vi "UpdateOutToFileFromFile.vi"(8 "ErrorArray In":errorcluster[](array[cluster]), 10 "TestFileRef In":T1, 11 "Bus In":refnum<class "Bus.lvclass">) -> (0 "ErrorArray Out":errorcluster[](array[cluster]), 2 "refnum out":T1, 3 "Bus Out":refnum<class "Bus.lvclass">)   [LabVIEW 2017, in "Bus_class.lvlib" / "Bus.lvclass"]
uses:
  Bus.lvclass
  <vilib>/Utility/config.llb/Config Data RefNum.ctl
  Modules/OutputToFilePlugins/OutputToFileBasePlugin/Typedefs/PmuCfgOpt.ctl
  TypeDefs/clBusData.ctl
  FrontPanel/TypeDefs/clEventConfig.ctl
  Modules/PmuImpairPlugins/PmuImpairPluginBase_class/TypeDefs/clImpairConfig.ctl
  Modules/EventPlugins/EventPluginBaseClass/TypeDefs/clEvtReportArray.ctl
  Modules/EventPlugins/EventPluginBaseClass/TypeDefs/clEvtReport.ctl
  Modules/EventPlugins/EventPluginBaseClass/TypeDefs/dblEvtSignalArray.ctl
  Modules/NetworkImpairmentModule/PublicAPI/Arguments/Broadcasts/dblNetworkTime.ctl
  Modules/NetworkImpairmentModule/PublicAPI/Arguments/Broadcasts/dblPktLoss.ctl
  Modules/FlagImpairModule/PublicAPI/Arguments/Broadcasts/ui32FlagImpairmentArray.ctl
  Modules/OutputToFilePlugins/OutputToFileBasePlugin/OutputToFileBasePlugin.lvclass
  Modules/FlagImpairModule/FlagImpairModule.lvlib
  Modules/NetworkImpairmentModule/NetworkImpairmentModule.lvlib
  Modules/EventPlugins/EventPluginBaseClass/EventPluginBaseClass.lvclass
  Modules/PmuImpairPlugins/PmuImpairPluginBase_class/PmuImpairPluginBase.lvclass
  Framework.lvlib
  <userlib>/NIST/NISTErrorLib/NISTErrorLib.lvlib
  <vilib>/Utility/config.llb/NI_LVConfig.lvlib
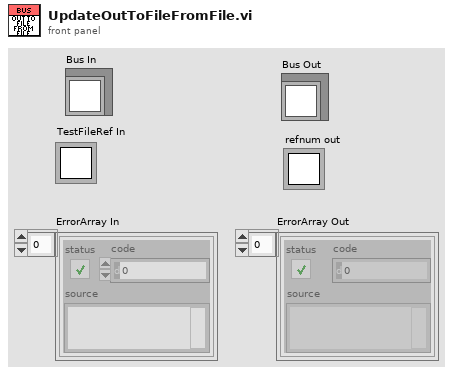
[diagram p1: front panel]
types:
  T1 = typedef "NI_LVConfig.lvlib/Config Data RefNum.ctl" = refnum<k1>
  T2 = typedef "Bus_class.lvlib/Bus.lvclass/clBusData.ctl" = cluster{"BusNumber":u8, "EvtPluginINIFilePath":path, "EvtParams":string[][], "EvtConfig":T3, "Start Time":dbl, "End Time":dbl, "PmuImpairPluginINIFilePath":path, "PmuImpairParams ":string[][], "PmuImpairConfig":T4, "NetImpPluginINIFilePath":path, "NetImpParams":string[][], "FlagImpPluginINIFilePath":path, "FlagImpParams":string[][], "EvtReportArray":T5, "EventSignalArray":T7, "ImpairReportArray":T5, "NetworkTime":T8, "PktLoss":T9, "FlagImpArray":T10, "OutputToFilePluginINIFilePath":path, "Output File Path":path, "clConfigOptions":T11, "AppPluginINIFilePath":path, "AppConfig":variant, "AppOutput":variant}
  T3 = typedef "Framework.lvlib/clEventConfig.ctl" = cluster{"UTC Time 0":timestamp, "Nominal Frequency":u16, "Reporting Rate":u16, "Fsamp":u32, "PosSeq":bool}
  T4 = typedef "PmuImpairPlugins.lvlib/PmuImpairPluginBase.lvclass/clImpairConfig.ctl" = cluster{"FilterType":string, "bPosSeq":bool}
  T5 = typedef "EventPlugins.lvlib/EventPluginBaseClass.lvclass/clEvtReportArray.ctl" = T6[]
  T6 = typedef "EventPlugins.lvlib/EventPluginBaseClass.lvclass/clEvtReport.ctl" = cluster{"Timestamp":dbl, "Synx":cdb[], "Freq":dbl, "ROCOF":dbl, "ID":i16}
  T7 = typedef "EventPlugins.lvlib/EventPluginBaseClass.lvclass/dblEvtSignalArray.ctl" = dbl[][]
  T8 = typedef "NetworkImpairmentModule.lvlib/dblNetworkTime.ctl" = dbl[]
  T9 = typedef "NetworkImpairmentModule.lvlib/dblPktLoss.ctl" = dbl[]
  T10 = typedef "FlagImpairModule.lvlib/ui32FlagImpairmentArray.ctl" = u32[]
  T11 = typedef "OutputToFilePlugins.lvlib/OutputToFileBasePlugin.lvclass/PmuCfgOpt.ctl" = cluster{"TIME_BASE":u64, "STN":string, "IDCODE":u16, "rdoPolRect":enum32{"Rectangular", "Polar"}, "rdoFloatInt":enum32{"Float", "Integer"}, "PHUNIT":u64, "rdoFreqDfreq":enum32{"Float", "Integer"}, "CHNAM":string[], "chkCfg2Prefix":bool}
  T12 = cluster{"OutputToFilePluginINIFilePath":path, "Output File Path":path, "clConfigOptions":T11}
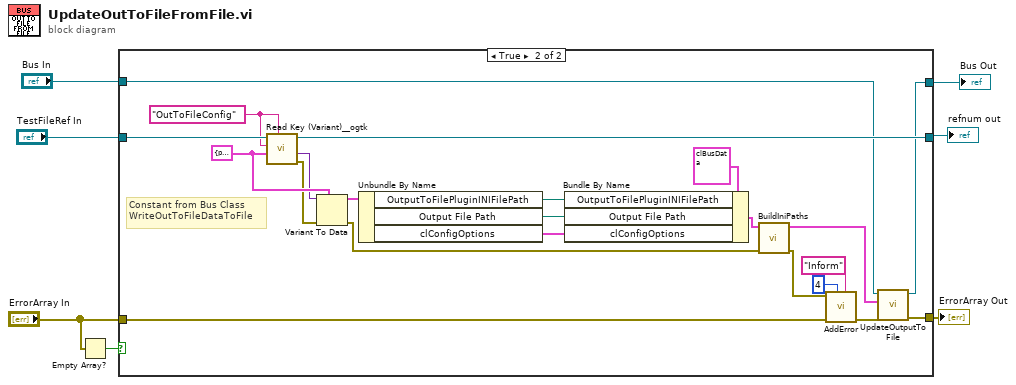
[diagram p0: block diagram]
diagram:
  n1 = Empty Array?(array="ErrorArray In") -> (empty?=w4:bool)
  n2 = case shown="True" w4 {
    tunnel: "TestFileRef In" -> [w10 w32]
    tunnel: "ErrorArray In" -> [w9 w21]
    tunnel: [w9 w19] -> w6
    tunnel: [w10 w18] -> w5
    tunnel: "Bus In" -> [w8 w17]
    tunnel: [w8 w16] -> w1
    frame False {
    }
    frame True {
      w29 = T12 {"OutputToFilePluginINIFilePath"=path "", "Output File Path"=path "", "clConfigOptions"={"TIME_BASE"=0, "STN"="", "IDCODE"=0, "rdoPolRect"=enum."Rectangular", "rdoFloatInt"=enum."Float", "PHUNIT"=0, "rdoFreqDfreq"=enum."Float", "CHNAM"=[], "chkCfg2Prefix"=FALSE}} ("output cluster")
      w31 = "OutToFileConfig" ("section")
      # "Constant from Bus Class\nWriteOutToFileDataToFile"
      n3 = call <userlib>:"Read Key (Variant)__ogtk.vi"("section"=w31, "type"=w29, "key (optional)"=w31, "refnum"=w32) -> ("error out"=w27:errorcluster, "key-value"=w28:variant, "refnum out"=w18:T1)  [unwired: 4 in, 1 out]
      n4 = Variant To Data(error in=w27, type=w29, Variant=w28) -> (data=w26:T12, error out=w11:errorcluster)
      n5 = Unbundle By Name(w26) -> ("OutputToFilePluginINIFilePath"=w15:path, "Output File Path"=w25:path, "clConfigOptions"=w24:T11)
      n6 = Bundle By Name(cluster=T2 {"BusNumber"=0, "EvtPluginINIFilePath"=path "", "EvtParams"=[], "EvtConfig"={"UTC Time 0"=timestamp(0 s since 1904-01-01), "Nominal Frequency"=60, "Reporting Rate"=60, "Fsamp"=960, "PosSeq"=FALSE}, "Start Time"=0.0, "End Time"=0.0, "PmuImpairPluginINIFilePath"=path "", "PmuImpairParams "=[["960"], ["8.19"], ["164"]], "PmuImpairConfig"={"FilterType"="", "bPosSeq"=TRUE}, "NetImpPluginINIFilePath"=path "", "NetImpParams"=[], "FlagImpPluginINIFilePath"=path "", "FlagImpParams"=[], "EvtReportArray"=[], "EventSignalArray"=[], "ImpairReportArray"=[], "NetworkTime"=[], "PktLoss"=[], "FlagImpArray"=[], "OutputToFilePluginINIFilePath"=path "", "Output File Path"=path "", "clConfigOptions"={"TIME_BASE"=1000000, "STN"="Bus_1", "IDCODE"=0, "rdoPolRect"=enum."Rectangular", "rdoFloatInt"=enum."Float", "PHUNIT"=1000000, "rdoFreqDfreq"=enum."Float", "CHNAM"=["VA", "VB", "VC", "V+", "IA", "IB", "IC", "I+"], "chkCfg2Prefix"=TRUE}, "AppPluginINIFilePath"=path "", "AppConfig"=variant, "AppOutput"=variant} ("clBusData"), "OutputToFilePluginINIFilePath"=w15, "Output File Path"=w25, "clConfigOptions"=w24) -> (w14:T2)
      n7 = call "BuildIniPaths.vi"("error in (no error)"=w11, "clBusData"=w14) -> ("error out"=w12:errorcluster, "clBusData"=w13:T2)  [unwired: 8 in]
      n8 = call <userlib>:"AddError.vi"("Severity"="Inform", "Priority"=u8 4, "ErrorArray"=w21, "error in (no error)"=w12) -> ("ErrorArray"=w20:errorcluster[])  [unwired: 6 in, 1 out]
      n9 = call "UpdateOutputToFile.vi"("ErrorArray In"=w20, "clBusData In"=w13, "Bus.lvclass In"=w17) -> ("ErrorArray Out"=w19:errorcluster[], "Bus.lvclass Out"=w16:refnum<class "Bus.lvclass">)  [unwired: 6 in, 1 out]
    }
  }
  "ErrorArray Out" <- w6
  "refnum out" <- w5
  "Bus Out" <- w1
